vi "Create Stub Files.vi"(8 "error in":errorcluster, 11 "Main Destination Path":path) -> (0 "error out":errorcluster)   [LabVIEW 2017, in "Build VIs.lvlib"]
uses:
  Build VIs.lvlib
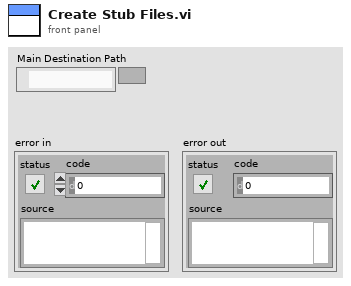
[diagram p1: front panel]
types:
  T1 = enum16{"open", "replace", "create", "open or create", "replace or create", "replace or create with confirmation"}
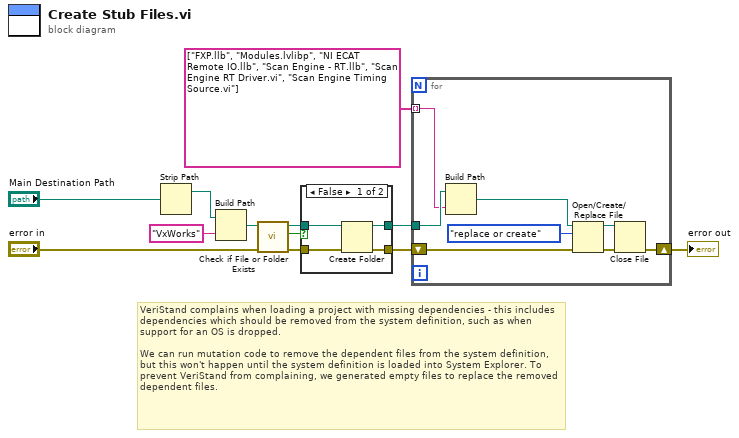
[diagram p0: block diagram]
diagram:
  # "VeriStand complains when loading a project with missing dependencies - this includes dependencies which should be removed from the system definition, such as when support for an OS is dropped.\n\nWe can run mutation code to remove the dependent files from the system definition, but this won't happen until the system definition is loaded into System Explorer. To prevent VeriStand from complaining, we generated empty files to replace the removed dependent files."
  n1 = Strip Path(path="Main Destination Path") -> (stripped path=w11:path)  [unwired: 1 out]
  n2 = Build Path(base path=w11, name or relative path="VxWorks") -> (appended path=w5:path)
  n3 = call <vilib>:"Check if File or Folder Exists.vi"("error in (no error)"="error in", "path"=w5) -> ("error out"=w2:errorcluster, "file or folder exists?"=w1:bool, "dup path"=w4:path)  [unwired: 7 in]
  n4 = case shown="False" w1 {
    tunnel: [w16 w18] -> w8
    tunnel: [w15 w17] -> w7
    tunnel: w4 -> [w14 w18]
    tunnel: w2 -> [w13 w17]
    frame False {
      n5 = Create Folder(path (use dialog)=w14, error in=w13) -> (created path=w16:path, error out=w15:errorcluster)  [unwired: 1 in, 1 out]
    }
    frame True {
    }
  }
  n6 = for {
    tunnel: w8 -> [w26]
    tunnel: string[] ["FXP.llb", "Modules.lvlibp", "NI ECAT Remote IO.llb", "Scan Engine - RT.llb", "Scan Engine RT Driver.vi", "Scan Engine Timing Source.vi"] ("name or relative path") -> [w25] mode=indexing
    shift-right: [w20] -> w6
    shift-left: w7 -> [w23]
    n7 = Build Path(base path=w26, name or relative path=w25) -> (appended path=w24:path)
    n8 = Open/Create/Replace File(file path (use dialog)=w24, error in=w23, operation (0:open)=T1."replace or create") -> (refnum out=w19:refnum<file>, error out=w22:errorcluster)  [unwired: 3 in, 1 out]
    n9 = Close File(refnum=w19, error in=w22) -> (error out=w20:errorcluster)  [unwired: 1 out]
  }
  "error out" <- w6
